vi "WPI_JoystickGetValues.vi"(8 "error in (no error)":errorcluster, 10 "Scaler":i8=127, 11 "JoystickDevRef":T1) -> (0 "error out":errorcluster, 1 "Buttons":bool[](array[boolean]), 2 "Axes":dbl[](array[numeric]), 3 "JoystickDevRef":T1, 4 "POVs":i16[](array[numeric]))   [LabVIEW 2017]
doc: "Returns button and scaled axis information about a joystick that you specify. \n\nThis software is licensed. Open the labview\\readme\\WPI Robotics Library Open Source License.txt file for more information."
uses:
  <vilib>/Rock Robotics/WPI/Joystick/WPI_JoystickDevRef.ctl
  <vilib>/Rock Robotics/WPI/Joystick/WPI_JoystickDeviceEnum.ctl
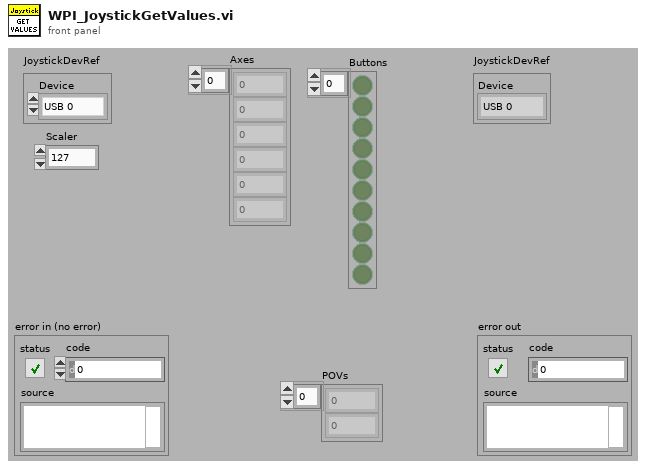
[diagram p1: front panel]
types:
  T1 = typedef "WPI_JoystickDevRef.ctl" = cluster{"Device":T2}
  T2 = typedef "WPI_JoystickDeviceEnum.ctl" = enum16{"USB 0", "USB 1", "USB 2", "USB 3", "USB 4", "USB 5"}
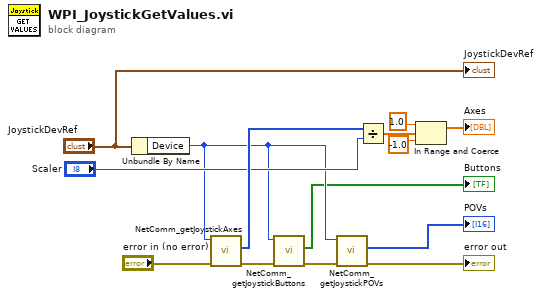
[diagram p0: block diagram]
diagram:
  n1 = Unbundle By Name("JoystickDevRef") -> ("Device"=w5:T2)
  n2 = call <vilib>:"NetComm_getJoystickAxes.vi"("error in (no error)"="error in (no error)", "Joystick Number"=w5) -> ("error out"=w10:errorcluster, "Axes"=w8:i16[])  [unwired: 8 in]
  n3 = call <vilib>:"NetComm_getJoystickButtons.vi"("error in (no error)"=w10, "Joystick Number"=w5) -> ("error out"=w9:errorcluster, "Buttons"=→"Buttons":bool[])  [unwired: 8 in]
  n4 = call <vilib>:"NetComm_getJoystickPOVs.vi"("error in (no error)"=w9, "Joystick Number"=w5) -> ("error out"=→"error out":errorcluster, "POVs"=→"POVs":i16[])  [unwired: 8 in]
  n5 = Divide(x=w8, y="Scaler") -> (x/y=w13:dbl[])
  n6 = In Range and Coerce(upper limit=1.0, x=w13, lower limit=-1.0) -> (coerced(x)=→"Axes":dbl[])  [unwired: 1 out]
  "JoystickDevRef" <- "JoystickDevRef"
